vi "Main RT.vi"(8 "Error In":errorcluster) -> (0 "Error Out":errorcluster)   [LabVIEW 2020]
uses:
  Control/FGV State.ctl
  Control/State - eFGV.ctl
panel:
  in  "stop":bool
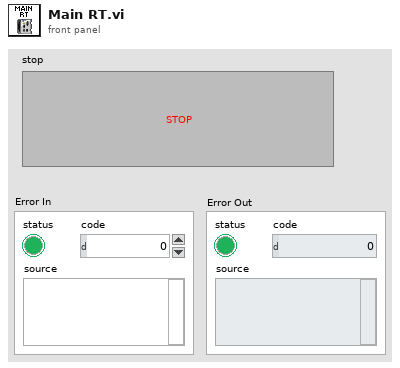
[diagram p1: front panel]
types:
  T1 = typedef "FGV State.ctl" = enum16{"Write", "Read"}
  T2 = typedef "State - eFGV.ctl" = enum16{"Init", "Read", "Write", "Exit"}
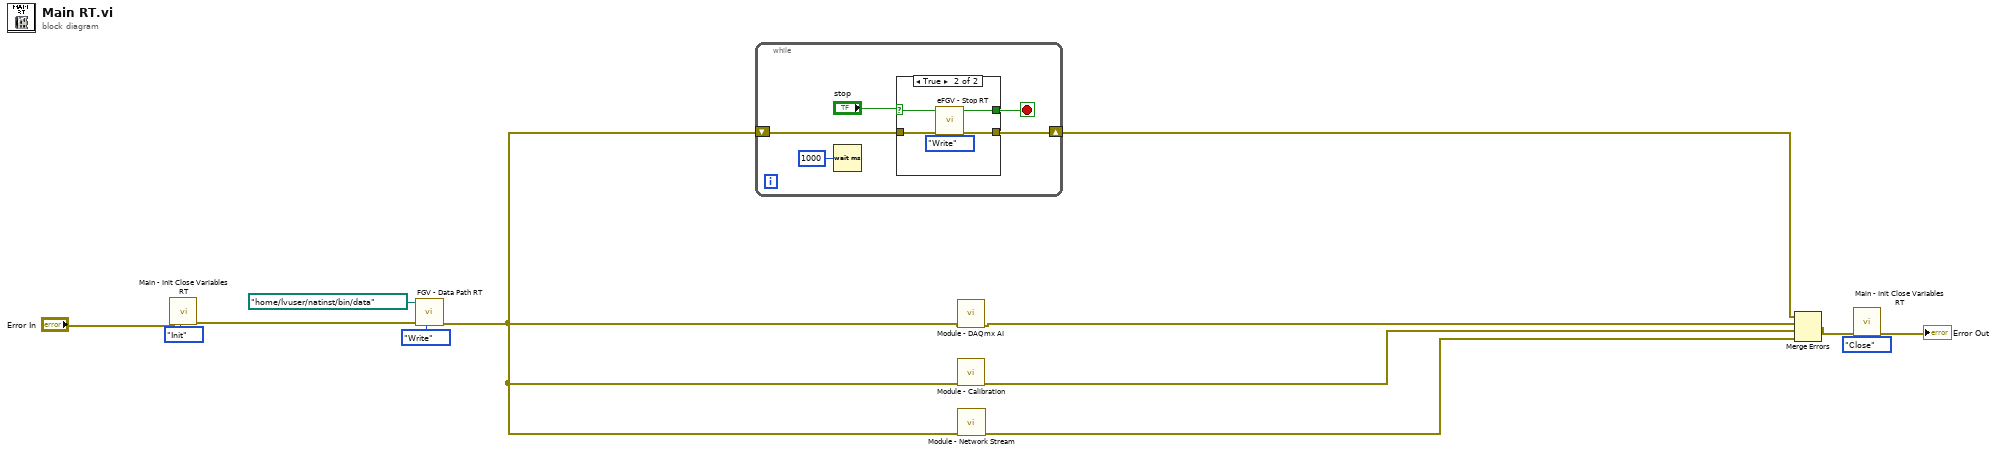
[diagram p0: block diagram]
diagram:
  n1 = call "Main - Init Close Variables RT.vi"("State"=enum16{"Init", "Close"}."Init", "Error In"="Error In") -> ("Error Out"=w4:errorcluster)  [unwired: 9 in]
  n2 = call "FGV - Data Path RT.vi"("FGV State"=FGV_State."Write", "Error In"=w4, "Path In"=path "/home/lvuser/natinst/bin/data") -> ("Error Out"=w3:errorcluster)  [unwired: 7 in, 1 out]
  n3 = while {
    shift-right: [w17] -> w2
    shift-left: w3 -> [w18]
    stop <- w16 stop-if-true
    n4 = Wait (ms)(milliseconds to wait=u32 1000) -> ()  [unwired: 1 out]
    n5 = case shown="True" "stop" {
      selector: "stop" -> [w19 w21]
      tunnel: w18 -> [w20 w25]
      tunnel: [w19 w22] -> w16
      tunnel: [w20 w24] -> w17
      frame False {
      }
      frame True {
        n6 = call "eFGV - Stop RT.vi"("State"=State_-_eFGV."Write", "Error In"=w25, "Stop RT? In"=w21) -> ("Error Out"=w24:errorcluster, "Stop RT? Out"=w22:bool)  [unwired: 6 in, 1 out]
      }
    }
  }
  n7 = call "Module - DAQmx AI.vi"("Error In"=w3) -> ("Error Out"=w8:errorcluster)  [unwired: 10 in]
  n8 = call "Module - Calibration.vi"("Error In"=w3) -> ("Error Out"=w9:errorcluster)  [unwired: 10 in]
  n9 = call "Module - Network Stream.vi"("error in (no error)"=w3) -> ("error out"=w10:errorcluster)  [unwired: 10 in]
  n10 = Merge Errors(w2, w8, w9, w10) -> (w12:errorcluster)
  n11 = call "Main - Init Close Variables RT.vi"("State"=enum16{"Init", "Close"}."Close", "Error In"=w12) -> ("Error Out"=→"Error Out":errorcluster)  [unwired: 9 in]
